vi "Configure BBM.vi"(7 "Config Folder":path, 8 "error in (no error)":errorcluster, 11 "WorkTable Class in":refnum<class "WorkTable Class.lvclass">) -> (0 "error out":errorcluster, 3 "WorkTable Class out":refnum<class "WorkTable Class.lvclass">)   [LabVIEW 2011, in "WorkTable Class.lvclass"]
uses:
  WorkTable Class.lvclass
  Type Definitions/Worktable_BBM Slot.ctl
  Vec3d Class/Vec3d Class.lvclass
  <vilib>/Utility/config.llb/Read Key (U32).vi
  <vilib>/Utility/config.llb/Read Key (String).vi
  <vilib>/Utility/config.llb/NI_LVConfig.lvlib
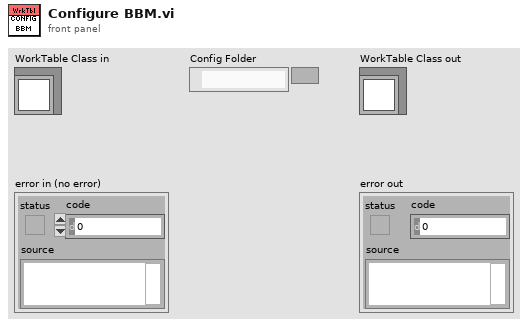
[diagram p1: front panel]
types:
  T1 = typedef "Worktable_BBM Slot.ctl" = cluster{"BBM Assembly State":enum16{"Empty", "Unglued", "Stamped", "PartOnTop", "Weighted"}, "BBM Type":enum16{"BBM", "GlassSlide"}, "HDI Type":enum16{"HDI", "Polyimide"}, "Fidicuals":refnum<class "Vec3d Class.lvclass">[], "Vacuum Channel":u8, "Boolean":bool}
  T2 = cluster{"BBM Chucks":cluster{"BBM Slots":T1[]}[]}
  T3 = enum16{"Empty", "Unglued", "Stamped", "PartOnTop", "Weighted"}
  T4 = typedef "NI_LVConfig.lvlib/Config Data RefNum.ctl" = refnum<k1>
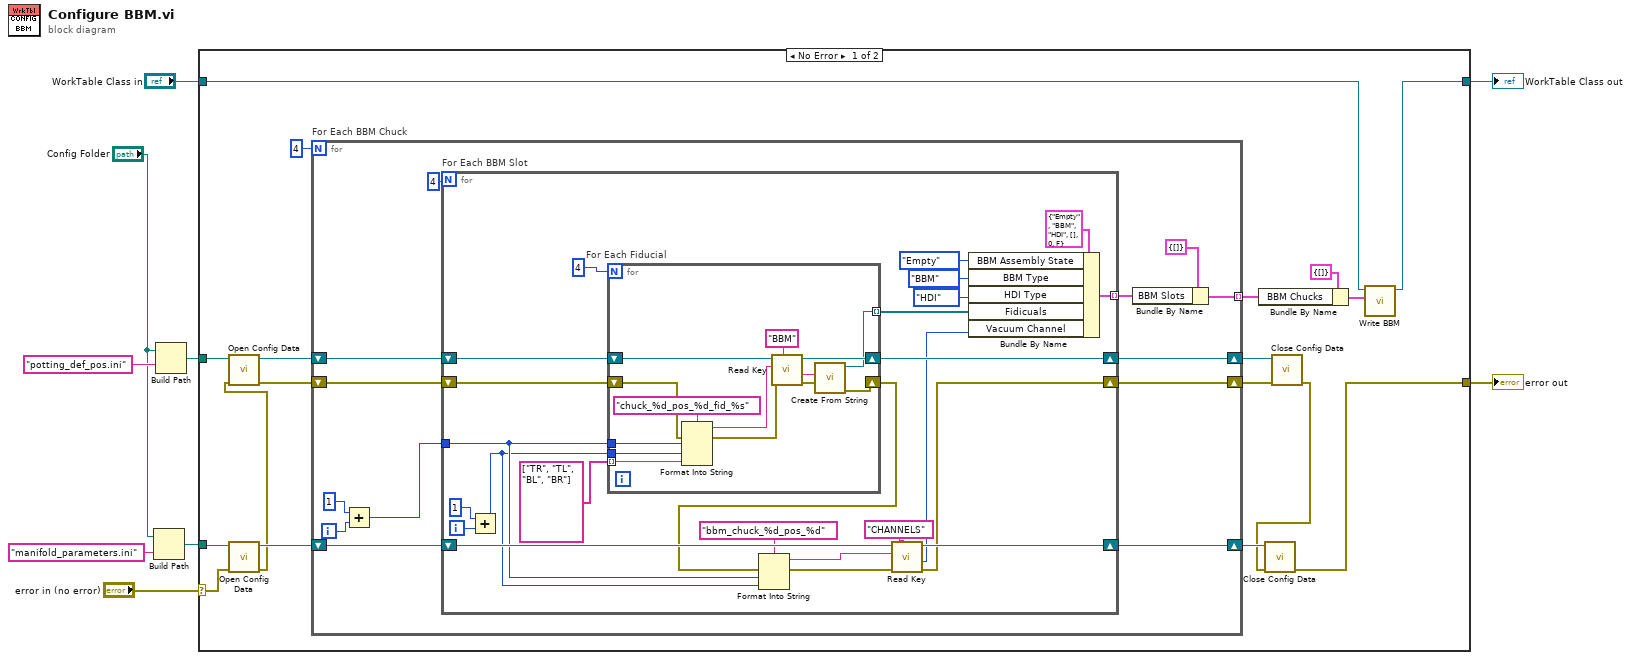
[diagram p0: block diagram]
diagram:
  n1 = Build Path(base path="Config Folder", name or relative path="manifold_parameters.ini") -> (appended path=w1:path)
  n2 = Build Path(base path="Config Folder", name or relative path="potting_def_pos.ini") -> (appended path=w4:path)
  n3 = case shown="No Error" "error in (no error)" {
    selector: "error in (no error)" -> [w18 w80]
    tunnel: [w14 w80] -> w8
    tunnel: "WorkTable Class in" -> [w20 w79]
    tunnel: [w19 w79] -> w6
    tunnel: w4 -> [w27 _]
    tunnel: w1 -> [w25 _]
    frame No Error {
      n4 = call <vilib>:"Open Config Data.vi"("error in (no error)"=w18, "configuration file path"=w25) -> ("error out"=w17:errorcluster, "refnum"=w24:T4)  [unwired: 7 in, 1 out]
      n5 = call <vilib>:"Open Config Data.vi"("error in (no error)"=w17, "configuration file path"=w27) -> ("error out"=w21:errorcluster, "refnum"=w22:T4)  [unwired: 7 in, 1 out]
      n6 = for "For Each BBM Chuck" {
        N: 4 -> [_]
        shift-right: [w38] -> w23
        shift-left: w22 -> [w33]
        shift-right: [w39] -> w26
        shift-left: w21 -> [w32]
        shift-right: [w31] -> w16
        shift-left: w24 -> [w37]
        tunnel: [w29] -> w10 mode=indexing
        i -> [w35]
        n7 = Add(x=1, y=w35) -> (x+y=w34:i32)
        n8 = for "For Each BBM Slot" {
          N: 4 ("dimension size") -> [_]
          tunnel: w34 -> [w48]
          shift-right: [w59] -> w38
          shift-left: w33 -> [w60]
          shift-right: [w44] -> w39
          shift-left: w32 -> [w61]
          tunnel: [w57] -> w28 mode=indexing
          shift-right: [w51] -> w31
          shift-left: w37 -> [w52]
          i -> [w58]
          n9 = Add(x=1, y=w58) -> (x+y=w47:i32)
          n10 = for "For Each Fiducial" {
            N: 4 -> [_]
            tunnel: string[] ["TR", "TL", "BL", "BR"] -> [w74] mode=indexing
            tunnel: w48 -> [w76]
            tunnel: w47 -> [w75]
            shift-right: [w65] -> w45
            shift-left: w61 -> [w70]
            shift-right: [w71] -> w59
            shift-left: w60 -> [w77]
            tunnel: [w66] -> w56 mode=indexing
            n11 = Format Into String(format string="chuck_%d_pos_%d_fid_%s", error in=w70, w76, w75, w74) -> (resulting string=w72:string, error out=w69:errorcluster)  [unwired: 1 in]
            n12 = call-poly <vilib>:"Read Key.vi"("section"="BBM", "error in (no error)"=w69, "key"=w72, "refnum"=w77) -> ("error out"=w68:errorcluster, "value"=w67:string, "refnum out"=w71:T4)  [unwired: 4 in, 1 out]
            n13 = call "Create From String.vi"("error in (no error)"=w68, "Input String"=w67) -> ("error out"=w65:errorcluster, "Vec3d Class out"=w66:refnum<class "Vec3d Class.lvclass">)  [unwired: 8 in]
          }
          n14 = Format Into String(format string="bbm_chuck_%d_pos_%d", error in=w45, w48, w47) -> (resulting string=w43:string, error out=w46:errorcluster)  [unwired: 1 in]
          n15 = call-poly <vilib>:"Read Key.vi"("section"="CHANNELS", "error in (no error)"=w46, "key"=w43, "refnum"=w52) -> ("error out"=w44:errorcluster, "value"=w42:u32, "refnum out"=w51:T4)  [unwired: 4 in, 1 out]
          n16 = Bundle By Name(cluster=T1 {"BBM Assembly State"=enum."Empty", "BBM Type"=enum."BBM", "HDI Type"=enum."HDI", "Fidicuals"=[], "Vacuum Channel"=0, "Boolean"=FALSE} ("element"), "BBM Assembly State"=T3."Empty", "BBM Type"=enum16{"BBM", "GlassSlide"}."BBM", "HDI Type"=enum16{"HDI", "Polyimide"}."HDI", "Fidicuals"=w56, "Vacuum Channel"=w42) -> (w57:T1)
        }
        n17 = Bundle By Name(cluster=cluster{"BBM Slots":T1[]} {"BBM Slots"=[]} ("element"), "BBM Slots"=w28) -> (w29:cluster{"BBM Slots":T1[]})
      }
      n18 = Bundle By Name(cluster=T2 {"BBM Chucks"=[]} ("BBM"), "BBM Chucks"=w10) -> (w11:T2)
      n19 = call <vilib>:"Close Config Data.vi"("error in (no error)"=w26, "refnum"=w23) -> ("error out"=w15:errorcluster)  [unwired: 8 in, 1 out]
      n20 = call <vilib>:"Close Config Data.vi"("error in (no error)"=w15, "refnum"=w16) -> ("error out"=w14:errorcluster)  [unwired: 8 in, 1 out]
      n21 = call-dynamic "Write BBM.vi"("BBM"=w11, "WorkTable Class in"=w20) -> ("WorkTable Class out"=w19:refnum<class "WorkTable Class.lvclass">)  [unwired: 8 in, 1 out]
    }
    frame Error {
    }
  }
  "WorkTable Class out" <- w6
  "error out" <- w8
